vi "Remove file name.vi"(11 "Input path":path) -> (3 "Path with file name removed":path)   [LabVIEW 2013]
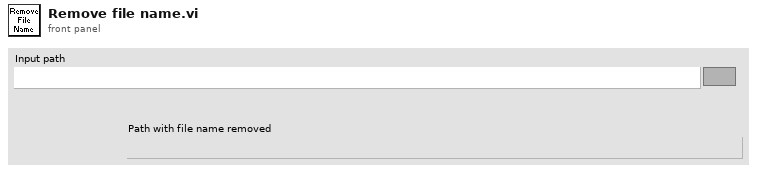
[diagram p1: front panel]
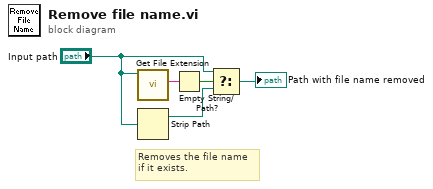
[diagram p0: block diagram]
diagram:
  # "Removes the file name\nif it exists."
  n1 = call <vilib>:"Get File Extension.vi"("file"="Input path") -> ("lowercase file extension"=w2:string)  [unwired: 7 in, 3 out]
  n2 = Strip Path(path="Input path") -> (stripped path=w5:path)  [unwired: 1 out]
  n3 = Empty String/Path?(string/path=w2) -> (empty?=w3:bool)
  n4 = Select(t="Input path", s=w3, f=w5) -> (s? t:f=→"Path with file name removed":path)
